vi "Open4TalonDrive.vi"   [LabVIEW 2016]
uses:
  <vilib>/Rock Robotics/WPI/ThirdParty/CanMotor/TalonSRX/WPI_CANTalonSRX_APIControlMode.ctl
  <vilib>/Rock Robotics/WPI/SafetyOutput/WPI_SafetyOutputConfigMenu.ctl
types:
  T1 = typedef "WPI_CANTalonSRX_APIControlMode.ctl" = enum8{"Percent VBus", "Speed", "Position", "Slave", "Unchanged / Invalid", "Voltage Compensation", "Current", "Motion Profile", "Motion Magic"}
  T2 = typedef "WPI_SafetyOutputConfigMenu.ctl" = enum16{"Enable", "Disable"}
  T3 = typedef "WPI_MotorControlDeviceRef.ctl" = cluster{"DeviceStatus":errorcluster, "Type":T4, "PWM":cluster{"PWM Channel":T5, "DeadBand":T6}, "CAN":cluster{"Device Number":u8, "SetOutput VI Ref":variant, "GetOutput VI Ref":variant, "Enable VI Ref":variant, "Disable VI Ref":variant, "Data":variant}, "Invert":bool}
  T4 = typedef "WPI_MotorControlType.ctl" = enum16{"PWM", "CAN"}
  T5 = typedef "FPGA_DIOPWMChannel.ctl" = enum8{"PWM 0", "PWM 1", "PWM 2", "PWM 3", "PWM 4", "PWM 5", "PWM 6", "PWM 7", "PWM 8", "PWM 9", "PWM MXP 0", "PWM MXP 1", "PWM MXP 2", "PWM MXP 3", "PWM MXP 4", "PWM MXP 5", "PWM MXP 6", "PWM MXP 7", "PWM MXP 8", "PWM MXP 9", "Invalid"}
  T6 = typedef "WPI_PWMDeadband.ctl" = cluster{"Name":string, "maxPositivePwm":i32, "minPositivePwm":i32, "centerPwm":i32, "maxNegativePwm":i32, "minNegativePwm":i32, "angularRange":u16}
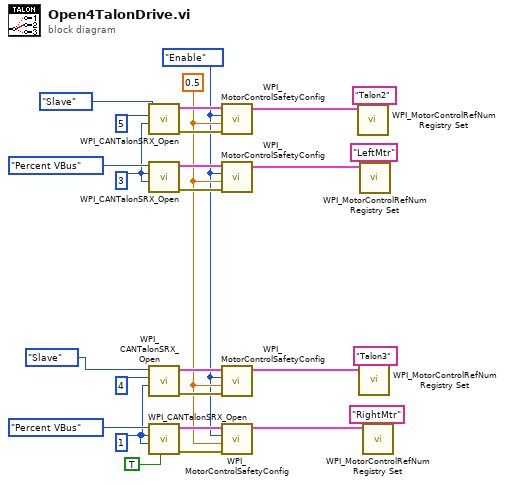
[diagram p0: block diagram]
diagram:
  w12 = WPI_SafetyOutputConfigMenu."Enable" ("mode")
  w9 = u8 1 ("Device Number")
  w13 = 0.5 ("timeout (s)")
  w8 = u8 3 ("Device Number")
  n1 = call <vilib>:"WPI_CANTalonSRX_Open.vi"("Master Device Number"=w8, "Device Number"=u8 5, "Control Mode"=WPI_CANTalonSRX_APIControlMode."Slave") -> ("error out"=w22:errorcluster, "CAN Talon SRX Ref"=w23:T3)  [unwired: 7 in]
  n2 = call <vilib>:"WPI_CANTalonSRX_Open.vi"("Master Device Number"=w8, "Device Number"=w8, "Control Mode"=WPI_CANTalonSRX_APIControlMode."Percent VBus") -> ("error out"=w24:errorcluster, "CAN Talon SRX Ref"=w25:T3)  [unwired: 7 in]
  n3 = call <vilib>:"WPI_CANTalonSRX_Open.vi"("Master Device Number"=w9, "Device Number"=u8 4, "Control Mode"=WPI_CANTalonSRX_APIControlMode."Slave") -> ("error out"=w15:errorcluster, "CAN Talon SRX Ref"=w16:T3)  [unwired: 7 in]
  n4 = call <vilib>:"WPI_CANTalonSRX_Open.vi"("Invert"=TRUE, "Master Device Number"=w9, "Device Number"=w9, "Control Mode"=WPI_CANTalonSRX_APIControlMode."Percent VBus") -> ("error out"=w17:errorcluster, "CAN Talon SRX Ref"=w18:T3)  [unwired: 6 in]
  n5 = call <vilib>:"WPI_MotorControlSafetyConfig.vi"("error in (no error)"=w22, "timeout (s)"=w13, "mode"=w12, "MotorControlDevRef"=w23) -> ("MotorControlDevRef"=w4:T3)  [unwired: 6 in, 1 out]
  n6 = call <vilib>:"WPI_MotorControlSafetyConfig.vi"("error in (no error)"=w24, "timeout (s)"=w13, "mode"=w12, "MotorControlDevRef"=w25) -> ("MotorControlDevRef"=w5:T3)  [unwired: 6 in, 1 out]
  n7 = call <vilib>:"WPI_MotorControlSafetyConfig.vi"("error in (no error)"=w15, "timeout (s)"=w13, "mode"=w12, "MotorControlDevRef"=w16) -> ("MotorControlDevRef"=w6:T3)  [unwired: 6 in, 1 out]
  n8 = call <vilib>:"WPI_MotorControlSafetyConfig.vi"("error in (no error)"=w17, "timeout (s)"=w13, "mode"=w12, "MotorControlDevRef"=w18) -> ("MotorControlDevRef"=w7:T3)  [unwired: 6 in, 1 out]
  n9 = call <vilib>:"WPI_MotorControlRefNum Registry Set.vi"("refnum name"="Talon2", "MotorControlDevRef"=w4) -> ()  [unwired: 8 in, 2 out]
  n10 = call <vilib>:"WPI_MotorControlRefNum Registry Set.vi"("refnum name"="Talon3", "MotorControlDevRef"=w6) -> ()  [unwired: 8 in, 2 out]
  n11 = call <vilib>:"WPI_MotorControlRefNum Registry Set.vi"("refnum name"="LeftMtr" ("Ref Name 1"), "MotorControlDevRef"=w5) -> ()  [unwired: 8 in, 2 out]
  n12 = call <vilib>:"WPI_MotorControlRefNum Registry Set.vi"("refnum name"="RightMtr" ("Ref Name 2"), "MotorControlDevRef"=w7) -> ()  [unwired: 8 in, 2 out]
